vi "VISJS Viewer.vi"(4 "Extra Scripts":string, 5 "FileDependency In":map{path, T1}(c390), 6 "Options":string, 7 "OpenWebBrowser(False)":bool, 8 "error in":errorcluster, 9 "Embedd VISJS Librarya in HTMl File(False)":bool, 10 "HTMLFilePath":path, 11 "LibraryDependency":map{path, T3}(c390)) -> (0 "error out":errorcluster, 3 "HTMLFileContent":string)   [LabVIEW 2020, in "VISJS Viewer.lvlib"] (continued)
else{var e=this._getNewTargetNode(A.x,A.y);this.body.nodes[e.id]=e,this.body.nodeIndices.push(e.id);var C=this.body.functions.createEdge({id:\"connectionEdge\"+rD(),from:A.id,to:e.id,physics:!1,smooth:{enabled:!0,type:\"continuous\",roundness:.5}});this.body.edges[C.id]=C,this.body.edgeIndices.push(C.id),this.temporaryIds.nodes.push(e.id),this.temporaryIds.edges.push(C.id)}this.touchTime=(new Date).valueOf()}}},{key:\"_dragControlNode\",value:function(g){var t=this.body.functions.getPointer(g.center),A=this.selectionHandler._pointerToPositionObject(t),e=void 0;void 0!==this.temporaryIds.edges[0]&&(e=this.body.edges[this.temporaryIds.edges[0]].fromId);for(var C=this.selectionHandler._getAllNodesOverlappingWith(A),I=void 0,i=C.length-1;i>=0;i--){var o;if(-1===Xc(o=this.temporaryIds.nodes).call(o,C[i])){I=this.body.nodes[C[i]];break}}if(g.controlEdge={from:e,to:I?I.id:void 0},this.selectionHandler.generateClickEvent(\"controlNodeDragging\",g,t),void 0!==this.temporaryIds.nodes[0]){var n=this.body.nodes[this.temporaryIds.nodes[0]];n.x=this.canvas._XconvertDOMtoCanvas(t.x),n.y=this.canvas._YconvertDOMtoCanvas(t.y),this.body.emitter.emit(\"_redraw\")}else this.interactionHandler.onDrag(g)}},{key:\"_finishConnect\",value:function(g){var t=this.body.functions.getPointer(g.center),A=this.selectionHandler._pointerToPositionObject(t),e=void 0;void 0!==this.temporaryIds.edges[0]&&(e=this.body.edges[this.temporaryIds.edges[0]].fromId);for(var C=this.selectionHandler._getAllNodesOverlappingWith(A),I=void 0,i=C.length-1;i>=0;i--){var o;if(-1===Xc(o=this.temporaryIds.nodes).call(o,C[i])){I=this.body.nodes[C[i]];break}}this._cleanupTemporaryNodesAndEdges(),void 0!==I&&(!0===I.isCluster?alert(this.options.locales[this.options.locale].createEdgeError||this.options.locales.en.createEdgeError):void 0!==this.body.nodes[e]&&void 0!==this.body.nodes[I.id]&&this._performAddEdge(e,I.id)),g.controlEdge={from:e,to:I?I.id:void 0},this.selectionHandler.generateClickEvent(\"controlNodeDragEnd\",g,t),this.body.emitter.emit(\"_redraw\")}},{key:\"_dragStartEdge\",value:function(g){var t=this.lastTouch;this.selectionHandler.generateClickEvent(\"dragStart\",g,t,void 0,!0)}},{key:\"_performAddNode\",value:function(g){var t=this,A={id:rD(),x:g.pointer.canvas.x,y:g.pointer.canvas.y,label:\"new\"};if(\"function\"==typeof this.options.addNode){if(2!==this.options.addNode.length)throw this.showManipulatorToolbar(),new Error(\"The function for add does not support two arguments (data,callback)\");this.options.addNode(A,(function(g){null!=g&&\"addNode\"===t.inMode&&t.body.data.nodes.getDataSet().add(g),t.showManipulatorToolbar()}))}else this.body.data.nodes.getDataSet().add(A),this.showManipulatorToolbar()}},{key:\"_performAddEdge\",value:function(g,t){var A=this,e={from:g,to:t};if(\"function\"==typeof this.options.addEdge){if(2!==this.options.addEdge.length)throw new Error(\"The function for connect does not support two arguments (data,callback)\");this.options.addEdge(e,(function(g){null!=g&&\"addEdge\"===A.inMode&&(A.body.data.edges.getDataSet().add(g),A.selectionHandler.unselectAll(),A.showManipulatorToolbar())}))}else this.body.data.edges.getDataSet().add(e),this.selectionHandler.unselectAll(),this.showManipulatorToolbar()}},{key:\"_performEditEdge\",value:function(g,t){var A=this,e={id:this.edgeBeingEditedId,from:g,to:t,label:this.body.data.edges.get(this.edgeBeingEditedId).label},C=this.options.editEdge;if(\"object\"===yd(C)&&(C=C.editWithoutDrag),\"function\"==typeof C){if(2!==C.length)throw new Error(\"The function for edit does not support two arguments (data, callback)\");C(e,(function(g){null==g||\"editEdge\"!==A.inMode?(A.body.edges[e.id].updateEdgeType(),A.body.emitter.emit(\"_redraw\"),A.showManipulatorToolbar()):(A.body.data.edges.getDataSet().update(g),A.selectionHandler.unselectAll(),A.showManipulatorToolbar())}))}else this.body.data.edges.getDataSet().update(e),this.selectionHandler.unselectAll(),this.showManipulatorToolbar()}}]),g}(),LM=\"string\",VM=\"boolean\",YM=\"number\",WM=\"array\",QM=\"object\",UM=[\"arrow\",\"bar\",\"box\",\"circle\",\"crow\",\"curve\",\"diamond\",\"image\",\"inv_curve\",\"inv_triangle\",\"triangle\",\"vee\"],_M={borderWidth:{number:YM},borderWidthSelected:{number:YM,undefined:\"undefined\"},brokenImage:{string:LM,undefined:\"undefined\"},chosen:{label:{boolean:VM,function:\"function\"},node:{boolean:VM,function:\"function\"},__type__:{object:QM,boolean:VM}},color:{border:{string:LM},background:{string:LM},highlight:{border:{string:LM},background:{string:LM},__type__:{object:QM,string:LM}},hover:{border:{string:LM},background:{string:LM},__type__:{object:QM,string:LM}},__type__:{object:QM,string:LM}},opacity:{number:YM,undefined:\"undefined\"},fixed:{x:{boolean:VM},y:{boolean:VM},__type__:{object:QM,boolean:VM}},font:{align:{string:LM},color:{string:LM},size:{number:YM},face:{string:LM},background:{string:LM},strokeWidth:{number:YM},strokeColor:{string:LM},vadjust:{number:YM},multi:{boolean:VM,string:LM},bold:{color:{string:LM},size:{number:YM},face:{string:LM},mod:{string:LM},vadjust:{number:YM},__type__:{object:QM,string:LM}},boldital:{color:{string:LM},size:{number:YM},face:{string:LM},mod:{string:LM},vadjust:{number:YM},__type__:{object:QM,string:LM}},ital:{color:{string:LM},size:{number:YM},face:{string:LM},mod:{string:LM},vadjust:{number:YM},__type__:{object:QM,string:LM}},mono:{color:{string:LM},size:{number:YM},face:{string:LM},mod:{string:LM},vadjust:{number:YM},__type__:{object:QM,string:LM}},__type__:{object:QM,string:LM}},group:{string:LM,number:YM,undefined:\"undefined\"},heightConstraint:{minimum:{number:YM},valign:{string:LM},__type__:{object:QM,boolean:VM,number:YM}},hidden:{boolean:VM},icon:{face:{string:LM},code:{string:LM},size:{number:YM},color:{string:LM},weight:{string:LM,number:YM},__type__:{object:QM}},id:{string:LM,number:YM},image:{selected:{string:LM,undefined:\"undefined\"},unselected:{string:LM,undefined:\"undefined\"},__type__:{object:QM,string:LM}},imagePadding:{top:{number:YM},right:{number:YM},bottom:{number:YM},left:{number:YM},__type__:{object:QM,number:YM}},label:{string:LM,undefined:\"undefined\"},labelHighlightBold:{boolean:VM},level:{number:YM,undefined:\"undefined\"},margin:{top:{number:YM},right:{number:YM},bottom:{number:YM},left:{number:YM},__type__:{object:QM,number:YM}},mass:{number:YM},physics:{boolean:VM},scaling:{min:{number:YM},max:{number:YM},label:{enabled:{boolean:VM},min:{number:YM},max:{number:YM},maxVisible:{number:YM},drawThreshold:{number:YM},__type__:{object:QM,boolean:VM}},customScalingFunction:{function:\"function\"},__type__:{object:QM}},shadow:{enabled:{boolean:VM},color:{string:LM},size:{number:YM},x:{number:YM},y:{number:YM},__type__:{object:QM,boolean:VM}},shape:{string:[\"custom\",\"ellipse\",\"circle\",\"database\",\"box\",\"text\",\"image\",\"circularImage\",\"diamond\",\"dot\",\"star\",\"triangle\",\"triangleDown\",\"square\",\"icon\",\"hexagon\"]},ctxRenderer:{function:\"function\"},shapeProperties:{borderDashes:{boolean:VM,array:WM},borderRadius:{number:YM},interpolation:{boolean:VM},useImageSize:{boolean:VM},useBorderWithImage:{boolean:VM},coordinateOrigin:{string:[\"center\",\"top-left\"]},__type__:{object:QM}},size:{number:YM},title:{string:LM,dom:\"dom\",undefined:\"undefined\"},value:{number:YM,undefined:\"undefined\"},widthConstraint:{minimum:{number:YM},maximum:{number:YM},__type__:{object:QM,boolean:VM,number:YM}},x:{number:YM},y:{number:YM},__type__:{object:QM}},KM={configure:{enabled:{boolean:VM},filter:{boolean:VM,string:LM,array:WM,function:\"function\"},container:{dom:\"dom\"},showButton:{boolean:VM},__type__:{object:QM,boolean:VM,string:LM,array:WM,function:\"function\"}},edges:{arrows:{to:{enabled:{boolean:VM},scaleFactor:{number:YM},type:{string:UM},imageHeight:{number:YM},imageWidth:{number:YM},src:{string:LM},__type__:{object:QM,boolean:VM}},middle:{enabled:{boolean:VM},scaleFactor:{number:YM},type:{string:UM},imageWidth:{number:YM},imageHeight:{number:YM},src:{string:LM},__type__:{object:QM,boolean:VM}},from:{enabled:{boolean:VM},scaleFactor:{number:YM},type:{string:UM},imageWidth:{number:YM},imageHeight:{number:YM},src:{string:LM},__type__:{object:QM,boolean:VM}},__type__:{string:[\"from\",\"to\",\"middle\"],object:QM}},endPointOffset:{from:{number:YM},to:{number:YM},__type__:{object:QM,number:YM}},arrowStrikethrough:{boolean:VM},background:{enabled:{boolean:VM},color:{string:LM},size:{number:YM},dashes:{boolean:VM,array:WM},__type__:{object:QM,boolean:VM}},chosen:{label:{boolean:VM,function:\"function\"},edge:{boolean:VM,function:\"function\"},__type__:{object:QM,boolean:VM}},color:{color:{string:LM},highlight:{string:LM},hover:{string:LM},inherit:{string:[\"from\",\"to\",\"both\"],boolean:VM},opacity:{number:YM},__type__:{object:QM,string:LM}},dashes:{boolean:VM,array:WM},font:{color:{string:LM},size:{number:YM},face:{string:LM},background:{string:LM},strokeWidth:{number:YM},strokeColor:{string:LM},align:{string:[\"horizontal\",\"top\",\"middle\",\"bottom\"]},vadjust:{number:YM},multi:{boolean:VM,string:LM},bold:{color:{string:LM},size:{number:YM},face:{string:LM},mod:{string:LM},vadjust:{number:YM},__type__:{object:QM,string:LM}},boldital:{color:{string:LM},size:{number:YM},face:{string:LM},mod:{string:LM},vadjust:{number:YM},__type__:{object:QM,string:LM}},ital:{color:{string:LM},size:{number:YM},face:{string:LM},mod:{string:LM},vadjust:{number:YM},__type__:{object:QM,string:LM}},mono:{color:{string:LM},size:{number:YM},face:{string:LM},mod:{string:LM},vadjust:{number:YM},__type__:{object:QM,string:LM}},__type__:{object:QM,string:LM}},hidden:{boolean:VM},hoverWidth:{function:\"function\",number:YM},label:{string:LM,undefined:\"undefined\"},labelHighlightBold:{boolean:VM},length:{number:YM,undefined:\"undefined\"},physics:{boolean:VM},scaling:{min:{number:YM},max:{number:YM},label:{enabled:{boolean:VM},min:{number:YM},max:{number:YM},maxVisible:{number:YM},drawThreshold:{number:YM},__type__:{object:QM,boolean:VM}},customScalingFunction:{function:\"function\"},__type__:{object:QM}},selectionWidth:{function:\"function\",number:YM},selfReferenceSize:{number:YM},selfReference:{size:{number:YM},angle:{number:YM},renderBehindTheNode:{boolean:VM},__type__:{object:QM}},shadow:{enabled:{boolean:VM},color:{string:LM},size:{number:YM},x:{number:YM},y:{number:YM},__type__:{object:QM,boolean:VM}},smooth:{enabled:{boolean:VM},type:{string:[\"dynamic\",\"continuous\",\"discrete\",\"diagonalCross\",\"straightCross\",\"horizontal\",\"vertical\",\"curvedCW\",\"curvedCCW\",\"cubicBezier\"]},roundness:{number:YM},forceDirection:{string:[\"horizontal\",\"vertical\",\"none\"],boolean:VM},__type__:{object:QM,boolean:VM}},title:{string:LM,undefined:\"undefined\"},width:{number:YM},widthConstraint:{maximum:{number:YM},__type__:{object:QM,boolean:VM,number:YM}},value:{number:YM,undefined:\"undefined\"},__type__:{object:QM}},groups:{useDefaultGroups:{boolean:VM},__any__:_M,__type__:{object:QM}},interaction:{dragNodes:{boolean:VM},dragView:{boolean:VM},hideEdgesOnDrag:{boolean:VM},hideEdgesOnZoom:{boolean:VM},hideNodesOnDrag:{boolean:VM},hover:{boolean:VM},keyboard:{enabled:{boolean:VM},speed:{x:{number:YM},y:{number:YM},zoom:{number:YM},__type__:{object:QM}},bindToWindow:{boolean:VM},autoFocus:{boolean:VM},__type__:{object:QM,boolean:VM}},multiselect:{boolean:VM},navigationButtons:{boolean:VM},selectable:{boolean:VM},selectConnectedEdges:{boolean:VM},hoverConnectedEdges:{boolean:VM},tooltipDelay:{number:YM},zoomView:{boolean:VM},zoomSpeed:{number:YM},__type__:{object:QM}},layout:{randomSeed:{undefined:\"undefined\",number:YM,string:LM},improvedLayout:{boolean:VM},clusterThreshold:{number:YM},hierarchical:{enabled:{boolean:VM},levelSeparation:{number:YM},nodeSpacing:{number:YM},treeSpacing:{number:YM},blockShifting:{boolean:VM},edgeMinimization:{boolean:VM},parentCentralization:{boolean:VM},direction:{string:[\"UD\",\"DU\",\"LR\",\"RL\"]},sortMethod:{string:[\"hubsize\",\"directed\"]},shakeTowards:{string:[\"leaves\",\"roots\"]},__type__:{object:QM,boolean:VM}},__type__:{object:QM}},manipulation:{enabled:{boolean:VM},initiallyActive:{boolean:VM},addNode:{boolean:VM,function:\"function\"},addEdge:{boolean:VM,function:\"function\"},editNode:{function:\"function\"},editEdge:{editWithoutDrag:{function:\"function\"},__type__:{object:QM,boolean:VM,function:\"function\"}},deleteNode:{boolean:VM,function:\"function\"},deleteEdge:{boolean:VM,function:\"function\"},controlNodeStyle:_M,__type__:{object:QM,boolean:VM}},nodes:_M,physics:{enabled:{boolean:VM},barnesHut:{theta:{number:YM},gravitationalConstant:{number:YM},centralGravity:{number:YM},springLength:{number:YM},springConstant:{number:YM},damping:{number:YM},avoidOverlap:{number:YM},__type__:{object:QM}},forceAtlas2Based:{theta:{number:YM},gravitationalConstant:{number:YM},centralGravity:{number:YM},springLength:{number:YM},springConstant:{number:YM},damping:{number:YM},avoidOverlap:{number:YM},__type__:{object:QM}},repulsion:{centralGravity:{number:YM},springLength:{number:YM},springConstant:{number:YM},nodeDistance:{number:YM},damping:{number:YM},__type__:{object:QM}},hierarchicalRepulsion:{centralGravity:{number:YM},springLength:{number:YM},springConstant:{number:YM},nodeDistance:{number:YM},damping:{number:YM},avoidOverlap:{number:YM},__type__:{object:QM}},maxVelocity:{number:YM},minVelocity:{number:YM},solver:{string:[\"barnesHut\",\"repulsion\",\"hierarchicalRepulsion\",\"forceAtlas2Based\"]},stabilization:{enabled:{boolean:VM},iterations:{number:YM},updateInterval:{number:YM},onlyDynamicEdges:{boolean:VM},fit:{boolean:VM},__type__:{object:QM,boolean:VM}},timestep:{number:YM},adaptiveTimestep:{boolean:VM},wind:{x:{number:YM},y:{number:YM},__type__:{object:QM}},__type__:{object:QM,boolean:VM}},autoResize:{boolean:VM},clickToUse:{boolean:VM},locale:{string:LM},locales:{__any__:{any:\"any\"},__type__:{object:QM}},height:{string:LM},width:{string:LM},__type__:{object:QM}},HM={nodes:{borderWidth:[1,0,10,1],borderWidthSelected:[2,0,10,1],color:{border:[\"color\",\"#2B7CE9\"],background:[\"color\",\"#97C2FC\"],highlight:{border:[\"color\",\"#2B7CE9\"],background:[\"color\",\"#D2E5FF\"]},hover:{border:[\"color\",\"#2B7CE9\"],background:[\"color\",\"#D2E5FF\"]}},opacity:[0,0,1,.1],fixed:{x:!1,y:!1},font:{color:[\"color\",\"#343434\"],size:[14,0,100,1],face:[\"arial\",\"verdana\",\"tahoma\"],background:[\"color\",\"none\"],strokeWidth:[0,0,50,1],strokeColor:[\"color\",\"#ffffff\"]},hidden:!1,labelHighlightBold:!0,physics:!0,scaling:{min:[10,0,200,1],max:[30,0,200,1],label:{enabled:!1,min:[14,0,200,1],max:[30,0,200,1],maxVisible:[30,0,200,1],drawThreshold:[5,0,20,1]}},shadow:{enabled:!1,color:\"rgba(0,0,0,0.5)\",size:[10,0,20,1],x:[5,-30,30,1],y:[5,-30,30,1]},shape:[\"ellipse\",\"box\",\"circle\",\"database\",\"diamond\",\"dot\",\"square\",\"star\",\"text\",\"triangle\",\"triangleDown\",\"hexagon\"],shapeProperties:{borderDashes:!1,borderRadius:[6,0,20,1],interpolation:!0,useImageSize:!1},size:[25,0,200,1]},edges:{arrows:{to:{enabled:!1,scaleFactor:[1,0,3,.05],type:\"arrow\"},middle:{enabled:!1,scaleFactor:[1,0,3,.05],type:\"arrow\"},from:{enabled:!1,scaleFactor:[1,0,3,.05],type:\"arrow\"}},endPointOffset:{from:[0,-10,10,1],to:[0,-10,10,1]},arrowStrikethrough:!0,color:{color:[\"color\",\"#848484\"],highlight:[\"color\",\"#848484\"],hover:[\"color\",\"#848484\"],inherit:[\"from\",\"to\",\"both\",!0,!1],opacity:[1,0,1,.05]},dashes:!1,font:{color:[\"color\",\"#343434\"],size:[14,0,100,1],face:[\"arial\",\"verdana\",\"tahoma\"],background:[\"color\",\"none\"],strokeWidth:[2,0,50,1],strokeColor:[\"color\",\"#ffffff\"],align:[\"horizontal\",\"top\",\"middle\",\"bottom\"]},hidden:!1,hoverWidth:[1.5,0,5,.1],labelHighlightBold:!0,physics:!0,scaling:{min:[1,0,100,1],max:[15,0,100,1],label:{enabled:!0,min:[14,0,200,1],max:[30,0,200,1],maxVisible:[30,0,200,1],drawThreshold:[5,0,20,1]}},selectionWidth:[1.5,0,5,.1],selfReferenceSize:[20,0,200,1],selfReference:{size:[20,0,200,1],angle:[Math.PI/2,-6*Math.PI,6*Math.PI,Math.PI/8],renderBehindTheNode:!0},shadow:{enabled:!1,color:\"rgba(0,0,0,0.5)\",size:[10,0,20,1],x:[5,-30,30,1],y:[5,-30,30,1]},smooth:{enabled:!0,type:[\"dynamic\",\"continuous\",\"discrete\",\"diagonalCross\",\"straightCross\",\"horizontal\",\"vertical\",\"curvedCW\",\"curvedCCW\",\"cubicBezier\"],forceDirection:[\"horizontal\",\"vertical\",\"none\"],roundness:[.5,0,1,.05]},width:[1,0,30,1]},layout:{hierarchical:{enabled:!1,levelSeparation:[150,20,500,5],nodeSpacing:[100,20,500,5],treeSpacing:[200,20,500,5],blockShifting:!0,edgeMinimization:!0,parentCentralization:!0,direction:[\"UD\",\"DU\",\"LR\",\"RL\"],sortMethod:[\"hubsize\",\"directed\"],shakeTowards:[\"leaves\",\"roots\"]}},interaction:{dragNodes:!0,dragView:!0,hideEdgesOnDrag:!1,hideEdgesOnZoom:!1,hideNodesOnDrag:!1,hover:!1,keyboard:{enabled:!1,speed:{x:[10,0,40,1],y:[10,0,40,1],zoom:[.02,0,.1,.005]},bindToWindow:!0,autoFocus:!0},multiselect:!1,navigationButtons:!1,selectable:!0,selectConnectedEdges:!0,hoverConnectedEdges:!0,tooltipDelay:[300,0,1e3,25],zoomView:!0,zoomSpeed:[1,.1,2,.1]},manipulation:{enabled:!1,initiallyActive:!1},physics:{enabled:!0,barnesHut:{theta:[.5,.1,1,.05],gravitationalConstant:[-2e3,-3e4,0,50],centralGravity:[.3,0,10,.05],springLength:[95,0,500,5],springConstant:[.04,0,1.2,.005],damping:[.09,0,1,.01],avoidOverlap:[0,0,1,.01]},forceAtlas2Based:{theta:[.5,.1,1,.05],gravitationalConstant:[-50,-500,0,1],centralGravity:[.01,0,1,.005],springLength:[95,0,500,5],springConstant:[.08,0,1.2,.005],damping:[.4,0,1,.01],avoidOverlap:[0,0,1,.01]},repulsion:{centralGravity:[.2,0,10,.05],springLength:[200,0,500,5],springConstant:[.05,0,1.2,.005],nodeDistance:[100,0,500,5],damping:[.09,0,1,.01]},hierarchicalRepulsion:{centralGravity:[.2,0,10,.05],springLength:[100,0,500,5],springConstant:[.01,0,1.2,.005],nodeDistance:[120,0,500,5],damping:[.09,0,1,.01],avoidOverlap:[0,0,1,.01]},maxVelocity:[50,0,150,1],minVelocity:[.1,.01,.5,.01],solver:[\"barnesHut\",\"forceAtlas2Based\",\"repulsion\",\"hierarchicalRepulsion\"],timestep:[.5,.01,1,.01],wind:{x:[0,-10,10,.1],y:[0,-10,10,.1]}}},XM=function(g,t,A){var e;return!(!Ic(g).call(g,\"physics\")||!Ic(e=HM.physics.solver).call(e,t)||A.physics.solver===t||\"wind\"===t)},JM=Object.freeze({__proto__:null,allOptions:KM,configuratorHideOption:XM,configureOptions:HM}),qM=function(){function g(){cn(this,g)}return kd(g,[{key:\"getDistances\",value:function(g,t,A){for(var e={},C=g.edges,I=0;I<t.length;I++){var i={};e[t[I]]=i;for(var o=0;o<t.length;o++)i[t[o]]=I==o?0:1e9}for(var n=0;n<A.length;n++){var r=C[A[n]];!0===r.connected&&void 0!==e[r.fromId]&&void 0!==e[r.toId]&&(e[r.fromId][r.toId]=1,e[r.toId][r.fromId]=1)}for(var s=t.length,a=0;a<s;a++)for(var d=t[a],h=e[d],l=0;l<s-1;l++)for(var c=t[l],u=e[c],p=l+1;p<s;p++){var f=t[p],v=e[f],y=Math.min(u[f],u[d]+h[f]);u[f]=y,v[c]=y}return e}}]),g}(),$M=function(){function g(t,A,e){cn(this,g),this.body=t,this.springLength=A,this.springConstant=e,this.distanceSolver=new qM}return kd(g,[{key:\"setOptions\",value:function(g){g&&(g.springLength&&(this.springLength=g.springLength),g.springConstant&&(this.springConstant=g.springConstant))}},{key:\"solve\",value:function(g,t){var A=arguments.length>2&&void 0!==arguments[2]&&arguments[2],e=this.distanceSolver.getDistances(this.body,g,t);this._createL_matrix(e),this._createK_matrix(e),this._createE_matrix();for(var C=0,I=Math.max(1e3,Math.min(10*this.body.nodeIndices.length,6e3)),i=1e9,o=0,n=0,r=0,s=0,a=0;i>.01&&C<I;){C+=1;var d=lh(this._getHighestEnergyNode(A),4);for(o=d[0],i=d[1],n=d[2],r=d[3],s=i,a=0;s>1&&a<5;){a+=1,this._moveNode(o,n,r);var h=lh(this._getEnergy(o),3);s=h[0],n=h[1],r=h[2]}}}},{key:\"_getHighestEnergyNode\",value:function(g){for(var t=this.body.nodeIndices,A=this.body.nodes,e=0,C=t[0],I=0,i=0,o=0;o<t.length;o++){var n=t[o];if(!0!==A[n].predefinedPosition||!0===A[n].isCluster&&!0===g||!0!==A[n].options.fixed.x||!0!==A[n].options.fixed.y){var r=lh(this._getEnergy(n),3),s=r[0],a=r[1],
